vi "XNET Bus Monitor Example.vi"() -> ()   [LabVIEW 2025, in "XNET Bus Monitor Client.lvlib"]
uses:
  XNET Bus Monitor Client.lvlib
  xnet_can_bus_monitor_api_client/RPC Messages/ni_xnet_can_bm_api_FrameFilter.ctl
  xnet_can_bus_monitor_api_client/RPC Messages/ni_xnet_can_bm_api_DirectionFilter.ctl
  Types/GUI.StateVariables.ctl
  Types/GUI.Controls.Refs.ctl
  Types/StreamEngine.QueueRefs.ctl
  Types/StreamEngine.CmdQueueData.ctl
  Types/StreamEngine.CmdQueueData.Cmd.ctl
  Types/SubProcessEngine.QueueRefs.ctl
  Types/SubProcessEngine.CmdQueueData.ctl
  Types/SubProcessEngine.CmdQueueData.Cmd.ctl
  Types/gRPC.ConnectionInfo.ctl
  <vilib>/gRPC/LabVIEW gRPC Library/Shared/grpcId.ctl
  Types/StreamEngine.State.ctl
  Types/SubProcessEngine.State.ctl
  Types/StreamEngine.CmdQueueData.InitialSettings.ctl
  xnet_can_bus_monitor_api_client/RPC Messages/ni_xnet_can_bm_api_StreamBusReply.ctl
  xnet_can_bus_monitor_api_client/RPC Messages/ni_xnet_can_bm_api_CanCommState.ctl
  xnet_can_bus_monitor_api_client/RPC Messages/ni_xnet_can_bm_api_CommState.ctl
  xnet_can_bus_monitor_api_client/RPC Messages/ni_xnet_can_bm_api_LastCommError.ctl
  xnet_can_bus_monitor_api_client/RPC Messages/ni_xnet_can_bm_api_Frame.ctl
  xnet_can_bus_monitor_api_client/RPC Messages/ni_xnet_can_bm_api_ErrorInfo.ctl
  Types/SubProcessEngine.CmdQueueData.Publish.ctl
  Types/StreamEngine.Parameters.ctl
  xnet_can_bus_monitor_api_client/RPC Messages/ni_xnet_can_bm_api_FilterInfo.ctl
  xnet_can_bus_monitor_api_client/RPC Messages/ni_xnet_can_bm_api_PassThruRequest.ctl
  xnet_can_bus_monitor_api_client/RPC Messages/ni_xnet_can_bm_api_SetStreamingFilterRequest.ctl
  <vilib>/Utility/miscctls.llb/LVRowAndColumnUnsignedTypeDef.ctl
  <vilib>/dlg_ctls.llb/Space Constant.vi
  SubVIs/Convert.BusDataArrayToStringArray.vi
  <vilib>/Utility/error.llb/Trim Whitespace.vi
  SubVIs/Convert.TimeToUTCString.vi
  <vilib>/Utility/error.llb/Trim Whitespace One-Sided.vi
  <vilib>/Utility/libraryn.llb/Check if File or Folder Exists.vi
  <vilib>/Utility/libraryn.llb/Get File Extension.vi
  <userlib>/_OpenG.lib/array/array.llb/Sort Array__ogtk.vi
  <userlib>/_OpenG.lib/array/array.llb/Sort 2D Array (String)__ogtk.vi
  xnet_can_bus_monitor_api_client/RPC Service/NI_XNET_CAN_Bus_Monitor_API/Begin NI_XNET_CAN_Bus_Monitor_API StreamBus.vi
  xnet_can_bus_monitor_api_client/RPC Service/NI_XNET_CAN_Bus_Monitor_API/End NI_XNET_CAN_Bus_Monitor_API StreamBus.vi
  xnet_can_bus_monitor_api_client/xnet_can_bus_monitor_api_client.lvlib
  <vilib>/gRPC/LabVIEW gRPC Library/grpc-lvsupport-release.lvlib
panel:
  out "error out":errorcluster
  out "Device":string
  in  "Tab Control":enum32{"Bus Stream", "RAW"}(tab)
  out "Log Status":string
  in  "Direction Filter":T1
  in  "Type Filter":T2
  in  "Reset Filter":bool
  in  "Host Filter":bool
  in  "Filter IDs":string caption="Filter IDs (format = x<ID>, comma separated, ID x0 = Bus Error)"
  in  "Clear History":bool
  out "Table Control":string[][](table)
  in  "Sort By ID":bool
  out "Stream Connected":bool
  out "Bus Status":string
  in  "Log":bool
  in  "Pause":bool
  in  "Extended?":bool
  in  "Identifier":u32 format="%x"
  in  "Raw Bytes":u8[](array[numeric])
  in  "Type":T3(ring)
  out "Error":errorcluster
  in  "Clear Raw":bool
  in  "Send Raw":bool
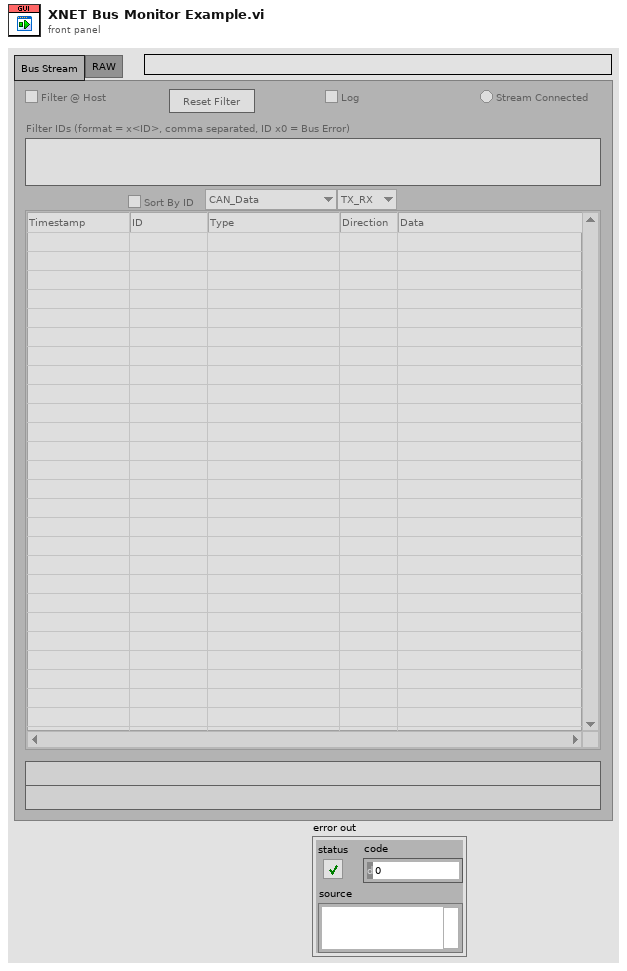
[diagram p1: front panel]
types:
  T1 = typedef "xnet_can_bus_monitor_api_client.lvlib/ni_xnet_can_bm_api_DirectionFilter.ctl" = enum32{"TX_RX", "RX", "TX"}
  T2 = typedef "xnet_can_bus_monitor_api_client.lvlib/ni_xnet_can_bm_api_FrameFilter.ctl" = enum32{"CAN_Data", "CAN_Remote", "CAN_Bus_Error", "CAN_2_Data", "CAN_FD_Data", "CAN_FD_BRS_Data", "J1939_Data", "Delay", "Log_Trigger", "Start_Trigger", "All"}
  T3 = enum16{"CAN Data", "CAN Remote", "CAN Bus Error", "CAN 2.0 Data", "CAN FD Data", "CAN FD+BRS Data", "J1939 Data", "Delay", "Log Trigger", "Start Trigger"}
  T4 = typedef "XNET Bus Monitor Client.lvlib/StreamEngine.CmdQueueData.InitialSettings.ctl" = cluster{"gRPC ID":T5, "Addon":string, "Project Folder":path}
  T5 = typedef "grpc-lvsupport-release.lvlib/grpcId.ctl" = u64
  T6 = typedef "XNET Bus Monitor Client.lvlib/SubProcessEngine.State.ctl" = enum8{"Idle", "Arm", "Process", "Stop", "Exit"}
  T7 = typedef "XNET Bus Monitor Client.lvlib/StreamEngine.State.ctl" = enum8{"Wait", "Start Stream", "Read Stream", "Stop Stream", "Exit"}
  T8 = typedef "XNET Bus Monitor Client.lvlib/GUI.StateVariables.ctl" = cluster{"UI.Refs":T9, "Connected?":bool, "Stream.Qs":T10, "Log Path":path, "gRPC Info":T12}
  T9 = typedef "XNET Bus Monitor Client.lvlib/GUI.Controls.Refs.ctl" = cluster{"Device":refnum<vi>, "Pause":refnum<vi>, "Table Control":refnum<vi>, "Sort By ID":refnum<vi>, "Streaming Connected":refnum<vi>, "Bus Status":refnum<vi>, "Direction Filter":refnum<vi>, "Type Filter":refnum<vi>, "Clear History":refnum<vi>, "Filter IDs":refnum<vi>, "Filter Location":refnum<vi>, "Reset Filter":refnum<vi>, "Log":refnum<vi>, "Type":refnum<vi>, "Extended?":refnum<vi>, "Identifier":refnum<vi>, "Raw Bytes":refnum<vi>, "Send Raw":refnum<vi>, "Clear Raw":refnum<vi>, "Raw Error":refnum<vi>, "Log Status":refnum<vi>}
  T10 = typedef "XNET Bus Monitor Client.lvlib/StreamEngine.QueueRefs.ctl" = cluster{"Cmd":refnum<queue>, "SubProcesses":T11}
  T11 = typedef "XNET Bus Monitor Client.lvlib/SubProcessEngine.QueueRefs.ctl" = cluster{"Process":refnum<queue>, "Log":refnum<queue>}
  T12 = typedef "XNET Bus Monitor Client.lvlib/gRPC.ConnectionInfo.ctl" = cluster{"IP Address":string, "Service Name":string, "Found Port":u64, "ID":T5}
  T13 = typedef "xnet_can_bus_monitor_api_client.lvlib/ni_xnet_can_bm_api_PassThruRequest.ctl" = cluster{"frame":T14}
  T14 = typedef "xnet_can_bus_monitor_api_client.lvlib/ni_xnet_can_bm_api_Frame.ctl" = cluster{"timestamp":dbl, "payload":u8[], "identifier":u32, "frame_type":u32, "extended":bool, "echo":bool}
  T15 = typedef "xnet_can_bus_monitor_api_client.lvlib/ni_xnet_can_bm_api_SetStreamingFilterRequest.ctl" = cluster{"filter_info":T16}
  T16 = typedef "xnet_can_bus_monitor_api_client.lvlib/ni_xnet_can_bm_api_FilterInfo.ctl" = cluster{"filter_ids":u32[], "direction_filter":T1, "frame_filter":T2}
  T17 = typedef "LVRowAndColumnUnsignedTypeDef.ctl" = cluster{"Row":u32, "Column":u32}
  T18 = typedef "xnet_can_bus_monitor_api_client.lvlib/ni_xnet_can_bm_api_StopProcessReply.ctl" = cluster{"stopped":bool, "error":T19}
  T19 = typedef "xnet_can_bus_monitor_api_client.lvlib/ni_xnet_can_bm_api_ErrorInfo.ctl" = errorcluster
  T20 = enum8{"Enabled", "Disabled", "Disabled and Grayed Out"}
  T21 = typedef "xnet_can_bus_monitor_api_client.lvlib/ni_xnet_can_bm_api_PassThruReply.ctl" = cluster{"error":T19}
  T22 = typedef "xnet_can_bus_monitor_api_client.lvlib/ni_xnet_can_bm_api_SetStreamingFilterReply.ctl" = cluster{"error":T19}
  T23 = typedef "xnet_can_bus_monitor_api_client.lvlib/ni_xnet_can_bm_api_ResetStreamingFilterReply.ctl" = cluster{"filter_info":T16, "error":T19}
  T24 = typedef "xnet_can_bus_monitor_api_client.lvlib/ni_xnet_can_bm_api_GetStreamingFilterReply.ctl" = cluster{"filter_info":T16, "error":T19}
  T25 = typedef "XNET Bus Monitor Client.lvlib/SubProcessEngine.CmdQueueData.Publish.ctl" = cluster{"Response Data":T26, "Success":bool}
  T26 = typedef "xnet_can_bus_monitor_api_client.lvlib/ni_xnet_can_bm_api_StreamBusReply.ctl" = cluster{"can_comm_state":T27, "frame":T14[], "error":T19}
  T27 = typedef "xnet_can_bus_monitor_api_client.lvlib/ni_xnet_can_bm_api_CanCommState.ctl" = cluster{"fault_code":i32, "fault":bool, "comm_state":T28, "last_comm_error":T29, "receive_error_counter":u32, "transmit_error_counter":u32, "transceiver_error":bool, "sleep":bool}
  T28 = typedef "xnet_can_bus_monitor_api_client.lvlib/ni_xnet_can_bm_api_CommState.ctl" = enum32{"Error_Active", "Error_Passive", "Bus_Off", "Init"}
  T29 = typedef "xnet_can_bus_monitor_api_client.lvlib/ni_xnet_can_bm_api_LastCommError.ctl" = enum32{"None", "Stuff", "Form", "ACK", "Bit1", "Bit0", "CRC"}
  T30 = typedef "XNET Bus Monitor Client.lvlib/SubProcessEngine.CmdQueueData.ctl" = cluster{"Cmd":T31, "Parameters":variant}
  T31 = typedef "XNET Bus Monitor Client.lvlib/SubProcessEngine.CmdQueueData.Cmd.ctl" = enum16{"Arm", "Publish", "Stop", "Exit"}
  T32 = typedef "XNET Bus Monitor Client.lvlib/StreamEngine.Parameters.ctl" = cluster{"Host Filter":bool, "Filter Parameters":T16, "Sort By ID":bool, "Pause":bool, "Clear History":bool}
  T33 = typedef "XNET Bus Monitor Client.lvlib/StreamEngine.CmdQueueData.ctl" = cluster{"Cmd":T34, "Parameters":variant}
  T34 = typedef "XNET Bus Monitor Client.lvlib/StreamEngine.CmdQueueData.Cmd.ctl" = enum8{"Start Stream", "Stop Stream", "Exit"}
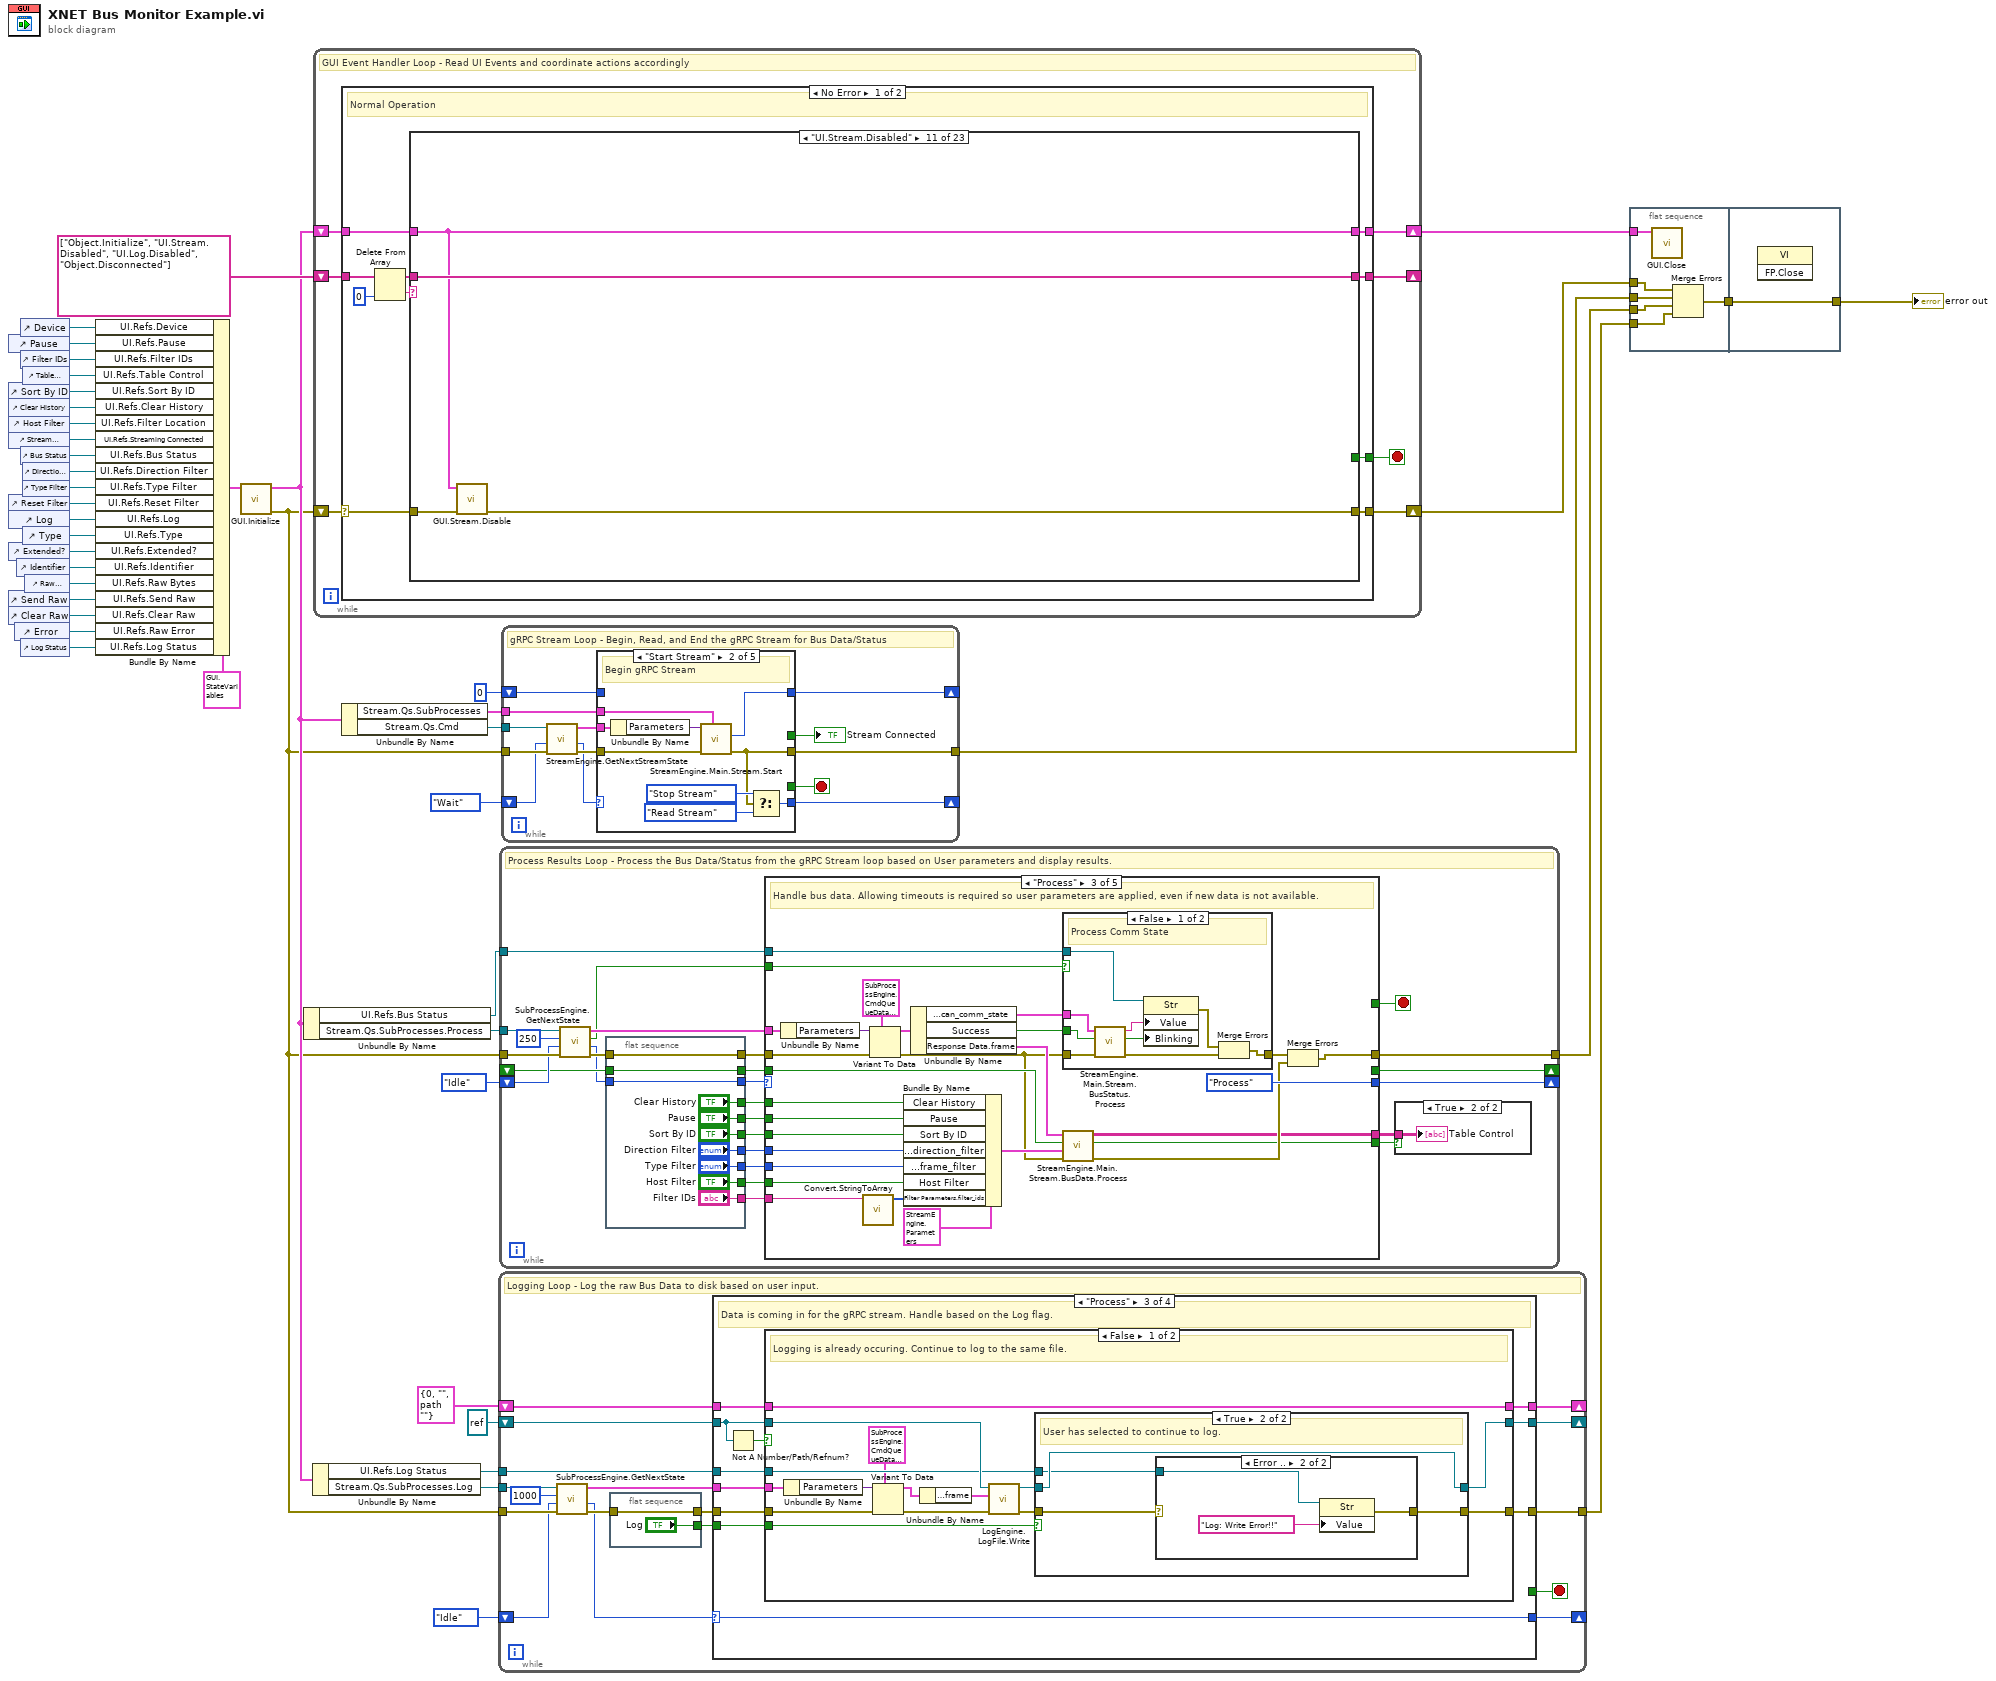
[diagram p0: block diagram]
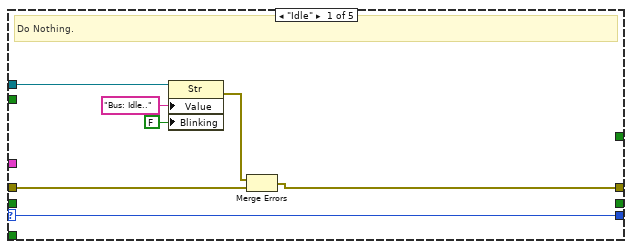
[diagram p3: hidden frame]
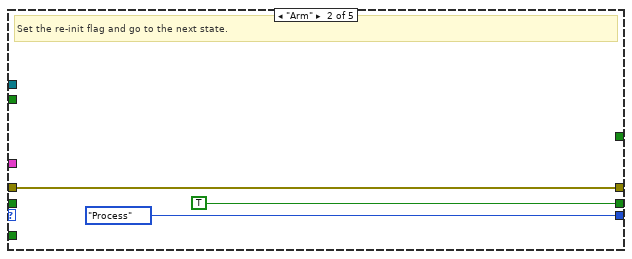
[diagram p4: hidden frame]
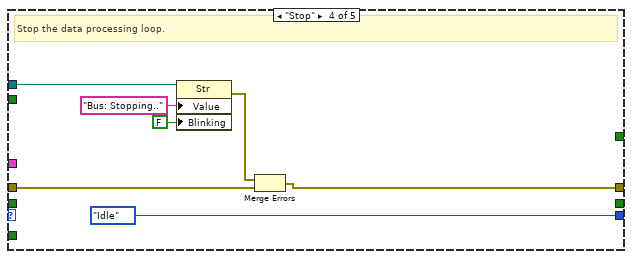
[diagram p6: hidden frame]
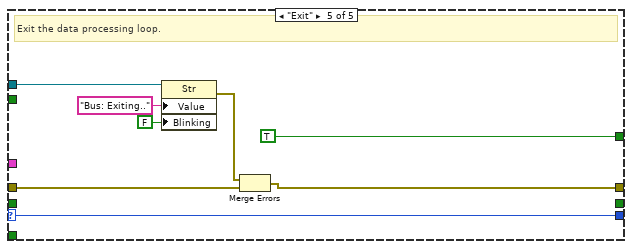
[diagram p7: hidden frame]
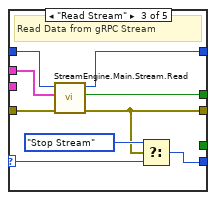
[diagram p9: hidden frame]
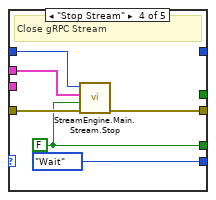
[diagram p10: hidden frame]
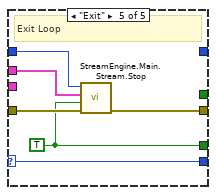
[diagram p11: hidden frame]
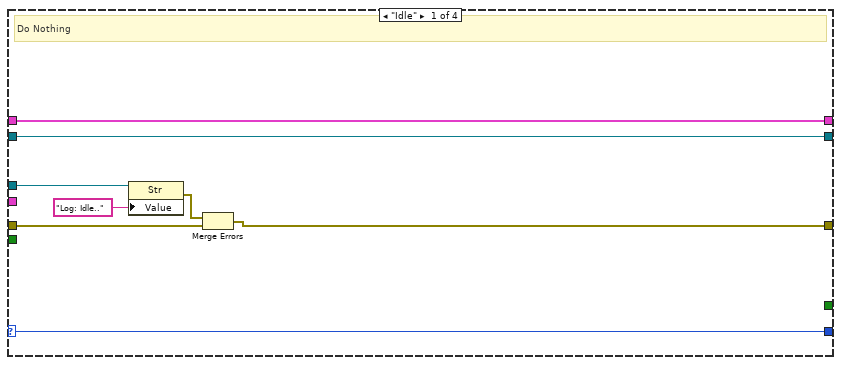
[diagram p12: hidden frame]
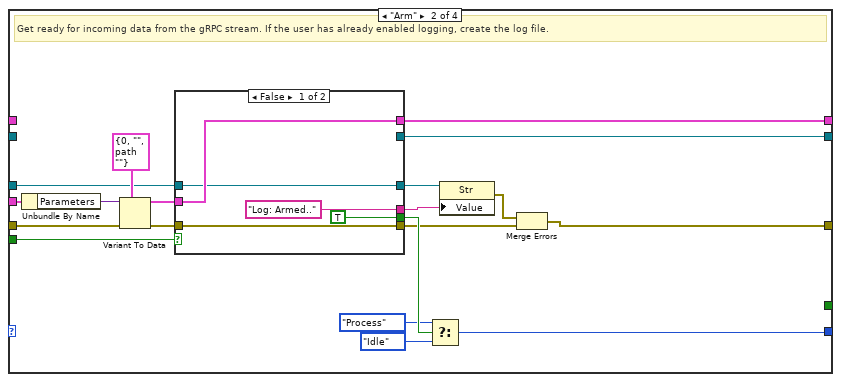
[diagram p13: hidden frame]
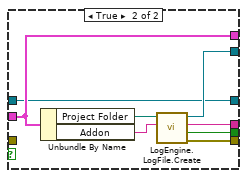
[diagram p14: hidden frame]
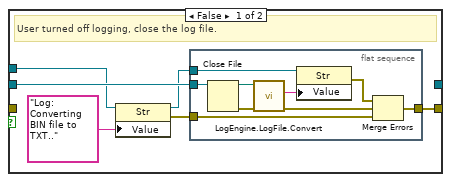
[diagram p15: hidden frame]
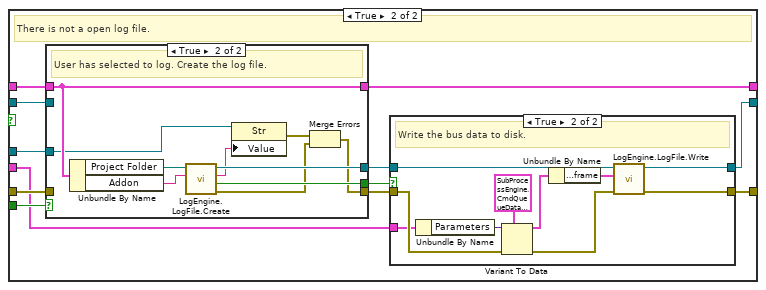
[diagram p17: hidden frame]
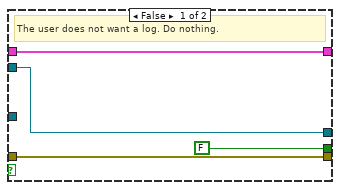
[diagram p19: hidden frame]
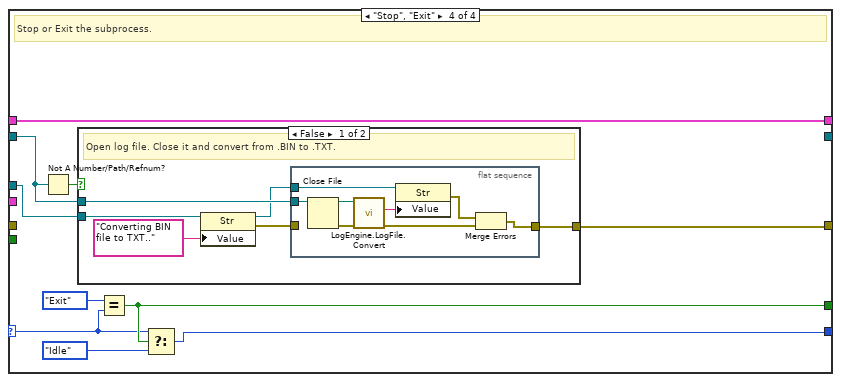
[diagram p20: hidden frame]
diagram:
  n1 = control-ref of="Pause"() -> (w22:refnum<vi>)
  n2 = control-ref of="Sort By ID"() -> (w41:refnum<vi>)
  n3 = control-ref of="Clear History"() -> (w37:refnum<vi>)
  n4 = control-ref of="Host Filter"() -> (w36:refnum<vi>)
  n5 = control-ref of="Stream Connected"() -> (w40:refnum<vi>)
  n6 = control-ref of="Reset Filter"() -> (w35:refnum<vi>)
  n7 = control-ref of="Log"() -> (w34:refnum<vi>)
  n8 = control-ref of="Extended?"() -> (w30:refnum<vi>)
  n9 = control-ref of="Send Raw"() -> (w27:refnum<vi>)
  n10 = control-ref of="Clear Raw"() -> (w28:refnum<vi>)
  n11 = control-ref of="Error"() -> (w29:refnum<vi>)
  n12 = control-ref of="Identifier"() -> (w31:refnum<vi>)
  n13 = control-ref of="Device"() -> (w24:refnum<vi>)
  n14 = control-ref of="Filter IDs"() -> (w38:refnum<vi>)
  n15 = control-ref of="Bus Status"() -> (w39:refnum<vi>)
  n16 = control-ref of="Log Status"() -> (w6:refnum<vi>)
  n17 = control-ref of="Table Control"() -> (w42:refnum<vi>)
  n18 = control-ref of="Direction Filter"() -> (w25:refnum<vi>)
  n19 = control-ref of="Type Filter"() -> (w26:refnum<vi>)
  n20 = control-ref of="Type"() -> (w33:refnum<vi>)
  n21 = control-ref of="Raw Bytes"() -> (w32:refnum<vi>)
  n22 = Bundle By Name(cluster=T8 {"UI.Refs"={"Device"=refnum, "Pause"=refnum, "Table Control"=refnum, "Sort By ID"=refnum, "Streaming Connected"=refnum, "Bus Status"=refnum, "Direction Filter"=refnum, "Type Filter"=refnum, "Clear History"=refnum, "Filter IDs"=refnum, "Filter Location"=refnum, "Reset Filter"=refnum, "Log"=refnum, "Type"=refnum, "Extended?"=refnum, "Identifier"=refnum, "Raw Bytes"=refnum, "Send Raw"=refnum, "Clear Raw"=refnum, "Raw Error"=refnum, "Log Status"=refnum}, "Connected?"=FALSE, "Stream.Qs"={"Cmd"=refnum, "SubProcesses"={"Process"=refnum, "Log"=refnum}}, "Log Path"=path "", "gRPC Info"={"IP Address"="", "Service Name"="", "Found Port"=0, "ID"=0}}, "UI.Refs.Device"=w24, "UI.Refs.Pause"=w22, "UI.Refs.Filter IDs"=w38, "UI.Refs.Table Control"=w42, "UI.Refs.Sort By ID"=w41, "UI.Refs.Clear History"=w37, "UI.Refs.Filter Location"=w36, "UI.Refs.Streaming Connected"=w40, "UI.Refs.Bus Status"=w39, "UI.Refs.Direction Filter"=w25, "UI.Refs.Type Filter"=w26, "UI.Refs.Reset Filter"=w35, "UI.Refs.Log"=w34, "UI.Refs.Type"=w33, "UI.Refs.Extended?"=w30, "UI.Refs.Identifier"=w31, "UI.Refs.Raw Bytes"=w32, "UI.Refs.Send Raw"=w27, "UI.Refs.Clear Raw"=w28, "UI.Refs.Raw Error"=w29, "UI.Refs.Log Status"=w6) -> (w23:T8)
  n23 = call "GUI.Initialize.vi"("State Variables in"=w23) -> ("error out"=w10:errorcluster, "State Variables out"=w13:T8)  [unwired: 9 in]
  n24 = Unbundle By Name(w13) -> ("UI.Refs.Bus Status"=w17:refnum<vi>, "Stream.Qs.SubProcesses.Process"=w18:refnum<queue>)
  n25 = Unbundle By Name(w13) -> ("UI.Refs.Log Status"=w5:refnum<vi>, "Stream.Qs.SubProcesses.Log"=w12:refnum<queue>)
  n26 = while {
    shift-right: [w50] -> _
    shift-left: string[] ["Object.Initialize", "UI.Stream.Disabled", "UI.Log.Disabled", "Object.Disconnected"] -> [w51]
    shift-right: [w48] -> w43
    shift-left: w13 -> [w47]
    shift-right: [w49] -> w8
    shift-left: w10 -> [w46]
    stop <- w52 stop-if-true
    # "GUI Event Handler Loop - Read UI Events and coordinate actions accordingly"
    n27 = case shown="No Error" w46 {
      selector: w46 -> [w53 w402]
      tunnel: [w62 _] -> w52
      tunnel: w51 -> [w60 w406]
      tunnel: [w57 w406] -> w50
      tunnel: [w56 w403] -> w49
      tunnel: [w55 w405] -> w48
      tunnel: w47 -> [w54 w405]
      frame No Error {
        # "Normal Operation"
        n28 = Delete From Array(array=w60, index=0) -> (deleted portion=w59:string, array with subset deleted=w58:string[])  [unwired: 1 in]
        n29 = case shown="\"UI.Stream.Disabled\"" w59 {
          tunnel: [_ _ _ _ _ _ _ _ _ _ _ _ _ _ _ _ _ _ _ _ _ FALSE TRUE] -> w62
          tunnel: [w65 w71 w170 w178 w227 w235 w258 w260 w267 w281 w294 w307 w324 w328 w336 w349 w357 w369 w380 w386 w391 w397 w401] -> w57
          tunnel: w53 -> [w64 w69 w166 w176 w224 w232 w256 w262 w265 w278 w292 w304 w323 w327 w335 w347 w355 w367 w378 w381 w387 w394 w398]
          tunnel: w58 -> [w65 w70 w170 w177 w227 w235 w258 w259 w267 w281 w294 w307 w324 w328 w336 w349 w357 w369 w380 w386 w391 w397 w401]
          tunnel: w54 -> [w63 w66 w169 w174 w225 w229 w255 w263 w264 w280 w293 w306 w322 w326 w333 w348 w356 w368 w379 w385 w390 w393 w399]
          tunnel: [w64 w68 w162 w175 w214 w231 w246 w262 w266 w269 w291 w296 w323 w327 w334 w347 w355 w367 w378 w382 w388 w395 w398] -> w56
          tunnel: [w63 w67 w169 w179 w221 w230 w250 w263 w264 w280 w293 w306 w322 w326 w333 w348 w356 w368 w379 w385 w390 w393 w399] -> w55
          frame Default {
            # "Do nothing."
          }
          frame "" {
            # "Check for new events."
            n30 = event shown="[1] \"Send Raw\": Value Change" {
              selector: _ -> [_ _ _ _ _ _ _ _ _ _]
              dyn-events: _ -> [_ _ _ _ _ _ _ _ _ _]
              timeout: 250 -> [_ _ _ _ _ _ _ _ _ _]
              tunnel: [w73 w78 w87 w99 w110 w119 w129 w142 w151 w158] -> w71
              tunnel: w70 -> [w73 w79 w88 w98 w109 w118 w128 w141 w152 w159]
              tunnel: w69 -> [w75 w80 w89 w100 w111 w120 w130 w143 w155 w161]
              tunnel: [w75 w80 w89 w100 w111 w120 w130 w143 w155 w161] -> w68
              tunnel: [w74 w77 w86 w97 w108 w117 w127 w140 w154 w160] -> w67
              tunnel: w66 -> [w74 w77 w86 w97 w108 w117 w127 w140 w154 w160]
              event Timeout {
                # "No new events to be handled. Do Nothing."
                n31 = event-data() -> ()  [unwired: 2 out]
              }
              event "Send Raw": Value Change {
                # "User entered a new raw message and is ready to Send."
                n32 = event-data() -> ()  [unwired: 2 out]
                n33 = Unbundle By Name(w77) -> ("Connected?"=w76:bool)
                n34 = case shown="True" w76 {
                  tunnel: w79 -> [w81 w83]
                  tunnel: [w81 w82] -> w78
                  frame False {
                  }
                  frame True {
                    n35 = Build Array (concatenate)(w83, string[] ["Raw.Send"]) -> (w82:string[])
                  }
                }
              }
              event "Clear Raw": Value Change {
                # "The user has selected to clear all the values in the Raw tab."
                n36 = event-data() -> ()  [unwired: 2 out]
                n37 = Unbundle By Name(w86) -> ("Connected?"=w85:bool)
                n38 = case shown="True" w85 {
                  tunnel: w88 -> [w90 w92]
                  tunnel: [w90 w91] -> w87
                  frame False {
                  }
                  frame True {
                    n39 = Build Array (concatenate)(w92, string[] ["Raw.Clear"]) -> (w91:string[])
                  }
                }
              }
              event "Filter IDs": Value Change {
                # "The user has changed which IDs to filter. Apply changes."
                n40 = event-data() -> ()  [unwired: 2 out]
                n41 = Unbundle By Name(w97) -> ("Connected?"=w95:bool)
                n42 = local read "Host Filter"() -> (w96:bool)
                n43 = Compound Arithmetic op=AND(invert w96, w95) -> (w94:bool)
                n44 = case shown="False" w94 {
                  tunnel: w98 -> [w101 w105]
                  tunnel: [w102 w104] -> w99
                  frame False {
                    # "Handle filtering on the client/host."
                    n45 = Build Array (concatenate)(w101, "Stream.Table.GoUp") -> (w102:string[])
                  }
                  frame True {
                    # "Send updated filter parameters to Server."
                    n46 = Build Array (concatenate)(w105, string[] ["Stream.Filter.Send", "Stream.Table.GoUp"]) -> (w104:string[])
                  }
                }
              }
              event "Clear History", "Sort By ID": Value Change {
                # "The user has selected to make table changes. The processing loop will handle this but make the table go to the top."
                n47 = event-data() -> ()  [unwired: 2 out]
                n48 = Unbundle By Name(w108) -> ("Connected?"=w107:bool)
                n49 = case shown="True" w107 {
                  tunnel: [w112 w115] -> w110
                  tunnel: w109 -> [w112 w114]
                  frame False {
                  }
                  frame True {
                    n50 = Build Array (concatenate)(w114, "Stream.Table.GoUp") -> (w115:string[])
                  }
                }
              }
              event "Reset Filter": Value Change {
                # "The user has reset which IDs to filter. Apply changes."
                n51 = event-data() -> ()  [unwired: 2 out]
                n52 = Unbundle By Name(w117) -> ("Connected?"=w116:bool)
                n53 = case shown="True" w116 {
                  tunnel: w118 -> [w121 w123]
                  tunnel: [w121 w122] -> w119
                  frame False {
                  }
                  frame True {
                    n54 = Build Array (concatenate)(w123, string[] ["Stream.Filter.Reset", "Stream.Table.GoUp"]) -> (w122:string[])
                  }
                }
              }
              event "Host Filter": Value Change {
                # "The user has changed where filtering happens. Apply changes."
                n55 = event-data() -> ("NewVal"=w125:bool)  [unwired: 1 out]
                n56 = Unbundle By Name(w127) -> ("Connected?"=w126:bool)
                n57 = case shown="True" w126 {
                  tunnel: w128 -> [w131 w134]
                  tunnel: [w131 w133] -> w129
                  tunnel: w125 -> [_ w132]
                  frame False {
                  }
                  frame True {
                    n58 = case shown="True" w132 {
                      tunnel: [string[] ["Stream.Filter.Send", "Stream.Table.GoUp"] string[] ["Stream.Filter.Clear", "Stream.Table.GoUp"]] -> w135
                      frame False {
                      }
                      frame True {
                      }
                    }
                    n59 = Build Array (concatenate)(w134, w135) -> (w133:string[])
                  }
                }
              }
              event "Log": Value Change {
                # "Log loop will handle the logging but force the GUI to latch the configuration while a log session is occuring."
                n60 = event-data() -> ("NewVal"=w138:bool)  [unwired: 1 out]
                n61 = Unbundle By Name(w140) -> ("Connected?"=w139:bool)
                n62 = case shown="True" w139 {
                  tunnel: w141 -> [w144 w147]
                  tunnel: [w144 w146] -> w142
                  tunnel: w138 -> [_ w145]
                  frame False {
                  }
                  frame True {
                    n63 = case shown="False" w145 {
                      tunnel: [string[] ["UI.Log.Disabled"] string[] ["UI.Log.Enabled"]] -> w148
                      frame False {
                      }
                      frame True {
                      }
                    }
                    n64 = Build Array (concatenate)(w147, w148) -> (w146:string[])
                  }
                }
              }
              event Menu Selection (User) {
                # "Queue up the Configure or Exit commands from the run time menu."
                n65 = event-data() -> ("ItemTag"=w153:string)  [unwired: 1 out]
                n66 = Build Array (concatenate)(w152, w153) -> (w151:string[])
              }
              event Panel Close? {
                # "Discard the user panel close and handle nicely."
                n67 = event-data() -> ()  [unwired: 5 out]
                n68 = Build Array (concatenate)(w159, "Object.Exit") -> (w158:string[])
                n69 = event-data("Discard?"=TRUE) -> ()  [unwired: 1 in, 1 out]
              }
            }
          }
          frame "Object.Initialize" {
            # "Initialize the GUI"
            n70 = Unbundle By Name(w169) -> ("UI.Refs.Device"=w164:refnum<vi>, "UI.Refs.Filter Location"=w167:refnum<vi>)
            n71 = property class="Bool (strict)"(reference=w167, error in=w166, "Value"=FALSE) -> (error out=w163:errorcluster)  [unwired: 1 out]
            n72 = local write "Tab Control"(0) -> ()
            n73 = property class="Str"(reference=w164, error in=w163, "Value"="Initializing!!") -> (error out=w162:errorcluster)  [unwired: 1 out]
          }
          frame "Object.Configure" {
            # "Allow the user to select a Port to display"
            n74 = Unbundle By Name(w174) -> ("gRPC Info.ID"=w173:T5)
            n75 = Equal To 0?(x=w173) -> (x = 0?=w172:bool)
            n76 = case shown="True" w172 {
              tunnel: [w181 w201] -> w179
              tunnel: [w180 w200] -> w178
              tunnel: w177 -> [w183 w199]
              tunnel: w176 -> [w187 w196]
              tunnel: [w187 w195] -> w175
              tunnel: w174 -> [w182 w192]
              frame False {
                # "A connection already exists. Ask the user if they want to close it."
                n77 = Two Button Dialog(message="Configuring will close the current session. Continue?", 2:"Yes" ("T button name (\"OK\")")) -> (T button?=w184:bool)  [unwired: 1 in]
                n78 = case shown="True" w184 {
                  tunnel: w183 -> [w188 _]
                  tunnel: w182 -> [w189 w191]
                  tunnel: [w189 w191] -> w181
                  tunnel: [w188 string[] ["Stream.Disable", "UI.Stream.Disabled", "UI.Log.Disabled", "Object.Disconnect", "Object.Disconnected", "Object.Initialize", "Object.Configure"]] -> w180
                  frame False {
                  }
                  frame True {
                  }
                }
              }
              frame True {
                # "No existing connection. Allow user to configure a new connection."
                n79 = call "GUI.ConfigureUI.vi"("error in (no error)"=w196) -> ("error out"=w194:errorcluster, "Log Path out"=w193:path, "Canceled?"=w198:bool, "gRPC Info"=w197:T12)  [unwired: 7 in]
                n80 = case shown="False" w198 {
                  tunnel: w192 -> [w204 w211]
                  tunnel: [w209 w211] -> w201
                  tunnel: [w207 w212] -> w200
                  tunnel: w199 -> [w208 w212]
                  tunnel: w197 -> [w205 _]
                  tunnel: [w203 w210] -> w195
                  tunnel: w194 -> [w203 w210]
                  tunnel: w193 -> [w202 _]
                  frame False {
                    n81 = Bundle By Name(cluster=w204, "gRPC Info"=w205, "Log Path"=w202) -> (w209:T8)
                    n82 = Build Array (concatenate)(w208, string[] ["Object.Initialize", "Stream.Disable", "UI.Stream.Disabled", "Stream.Enable", "UI.Stream.Enabled", "UI.Log.Enabled", "Object.Connected"]) -> (w207:string[])
                  }
                  frame True {
                    # "User canceled"
                  }
                }
              }
            }
          }
          frame "Object.Connected" {
            # "gRPC connected. Update the GUI accordingly."
            n83 = call "GUI.DisableState.Set.vi"("Enable?"=TRUE, "error in (no error)"=w224, "State Variables in"=w225) -> ("error out"=w220:errorcluster, "State Variables out"=w222:T8)  [unwired: 7 in]
            n84 = Unbundle By Name(w222) -> ("UI.Refs.Log"=w216:refnum<vi>, "Log Path"=w217:path, "UI.Refs.Device"=w219:refnum<vi>, "gRPC Info.Service Name"=w218:string)
            n85 = property class="Str"(reference=w219, error in=w220, "Value"=w218) -> (error out=w215:errorcluster)  [unwired: 1 out]
            n86 = call <vilib>:"Is Path and Not Empty.vi"("path"=w217) -> ("Is Path and Not Empty?"=w213:bool)  [unwired: 4 in]
            n87 = property class="Bool (strict)"(reference=w216, error in=w215, "Visible"=w213) -> (error out=w214:errorcluster)  [unwired: 1 out]
            n88 = Bundle By Name(cluster=w222, "Connected?"=TRUE) -> (w221:T8)
          }
          frame "Object.Disconnect" {
            # "Disconnect from the Server."
            n89 = Unbundle By Name(w229) -> ("gRPC Info.ID"=w233:T5)
            n90 = Equal To 0?(x=w233) -> (x = 0?=w234:bool)
            n91 = case shown="False" w234 {
              tunnel: w233 -> [w242 _]
              tunnel: w232 -> [w239 w244]
              tunnel: [w239 w244] -> w231
              frame False {
                n92 = call "NI_XNET_CAN_Bus_Monitor_API StopProcess.vi"("gRPC ID"=w242) -> ("error out"=w237:errorcluster, "Response Data"=w238:T18, "gRPC ID out"=w243:T5)  [unwired: 8 in]
                n93 = call "gRPC.Response.GetError.vi"("error in (no error)"=w237, "Response"=w238) -> ("error out"=w236:errorcluster)  [unwired: 9 in]
                n94 = call "Destroy Client.vi"("gRPC ID"=w243) -> ("error out"=w241:errorcluster)  [unwired: 10 in]
                n95 = Merge Errors(w236, w241) -> (w240:errorcluster)
                n96 = call <vilib>:"Simple Error Handler.vi"("error in (no error)"=w240) -> ()  [unwired: 4 in, 5 out]
              }
              frame True {
              }
            }
            n97 = Bundle By Name(cluster=w229, "gRPC Info"=T12 {"IP Address"="", "Service Name"="", "Found Port"=0, "ID"=0}) -> (w230:T8)
          }
          frame "Object.Disconnected" {
            # "Disconnected from the Server. Update the GUI accordingly."
            n98 = call "GUI.DisableState.Set.vi"("Enable?"=FALSE, "error in (no error)"=w256, "State Variables in"=w255) -> ("error out"=w252:errorcluster, "State Variables out"=w251:T8)  [unwired: 7 in]
            n99 = Unbundle By Name(w251) -> ("UI.Refs.Log"=w248:refnum<vi>, "UI.Refs.Device"=w253:refnum<vi>)
            n100 = property class="Str"(reference=w253, error in=w252, "Value"="Object Disconnected - Configure") -> (error out=w247:errorcluster)  [unwired: 1 out]
            n101 = property class="Bool (strict)"(reference=w248, error in=w247, "Visible"=TRUE ("Value")) -> (error out=w246:errorcluster)  [unwired: 1 out]
            n102 = Bundle By Name(cluster=w251, "Connected?"=FALSE) -> (w250:T8)
          }
          frame "Object.Exit" {
            # "Queue all the commands to cleanly exit."
            n103 = Build Array (concatenate)(w259, string[] ["Stream.Disable", "UI.Stream.Disabled", "UI.Log.Disabled", "Object.Disconnect", "Object.Disconnected", "Stream.Exit", "App.Exit"]) -> (w260:string[])
          }
          frame "UI.Stream.Enabled" {
            n104 = call "GUI.Stream.Enable.vi"("error in (no error)"=w265, "State Variables in"=w264) -> ("error out"=w266:errorcluster)  [unwired: 9 in]
          }
          frame "UI.Log.Enabled" {
            w268 = T20."Disabled and Grayed Out" ("Disabled")
            # "Logging has be enabled. Stop the user from changing filter settings so that the data coming from the Server is the same."
            n105 = Unbundle By Name(w280) -> ("UI.Refs.Type Filter"=w273:refnum<vi>, "UI.Refs.Filter IDs"=w272:refnum<vi>, "UI.Refs.Direction Filter"=w271:refnum<vi>, "UI.Refs.Reset Filter"=w276:refnum<vi>, "UI.Refs.Filter Location"=w279:refnum<vi>)
            n106 = property class="Bool (strict)"(reference=w279, error in=w278, "DisabledEnum"=w268) -> (error out=w277:errorcluster, "Value"=w275:bool)  [unwired: 1 out]
            n107 = Build Array(w273, w272, w271) -> (w270:refnum<vi>[])
            n108 = property class="Bool"(reference=w276, error in=w277, "DisabledEnum"=w268) -> (error out=w274:errorcluster)  [unwired: 1 out]
            n109 = case shown="False" w275 {
              tunnel: w274 -> [w284 w290]
              tunnel: w270 -> [w285 _]
              tunnel: [w283 w290] -> w269
              tunnel: w268 -> [w282 _]
              frame False {
                n110 = for {
                  tunnel: w285 -> [w289] mode=indexing
                  shift-right: [w287] -> w283
                  shift-left: w284 -> [w288]
                  tunnel: w282 -> [w286]
                  n111 = property class="Ctl"(reference=w289, error in=w288, "DisabledEnum"=w286) -> (error out=w287:errorcluster)  [unwired: 1 out]
                }
              }
              frame True {
              }
            }
          }
          frame "UI.Stream.Disabled" {
            n112 = call "GUI.Stream.Disable.vi"("error in (no error)"=w292, "State Variables in"=w293) -> ("error out"=w291:errorcluster)  [unwired: 9 in]
          }
          frame "UI.Log.Disabled" {
            w295 = T20."Enabled" ("Disabled")
            # "Logging has been turned off so re-enable the filter options."
            n113 = Unbundle By Name(w306) -> ("UI.Refs.Type Filter"=w300:refnum<vi>, "UI.Refs.Filter IDs"=w299:refnum<vi>, "UI.Refs.Direction Filter"=w298:refnum<vi>, "UI.Refs.Reset Filter"=w302:refnum<vi>, "UI.Refs.Filter Location"=w305:refnum<vi>)
            n114 = property class="Bool (strict)"(reference=w305, error in=w304, "DisabledEnum"=w295) -> (error out=w303:errorcluster)  [unwired: 1 out]
            n115 = Build Array(w300, w299, w298) -> (w297:refnum<vi>[])
            n116 = property class="Bool"(reference=w302, error in=w303, "DisabledEnum"=w295) -> (error out=w301:errorcluster)  [unwired: 1 out]
            n117 = for {
              tunnel: w297 -> [w311] mode=indexing
              shift-right: [w309] -> w296
              shift-left: w301 -> [w310]
              tunnel: w295 -> [w308]
              n118 = property class="Ctl"(reference=w311, error in=w310, "DisabledEnum"=w308) -> (error out=w309:errorcluster)  [unwired: 1 out]
            }
          }
          frame "Raw.Send" {
            # "Send a raw frame to be put directly on the bus."
            n119 = Bundle By Name(cluster=T13 {"frame"={"timestamp"=0.0, "payload"=[], "identifier"=0, "frame_type"=0, "extended"=FALSE, "echo"=FALSE}} ("Request Data"), "frame.extended"="Extended?", "frame.frame_type"="Type", "frame.identifier"="Identifier", "frame.payload"="Raw Bytes") -> (w316:T13)
            n120 = Unbundle By Name(w322) -> ("gRPC Info.ID"=w315:T5)
            n121 = call "NI_XNET_CAN_Bus_Monitor_API PassThru.vi"("Request Data"=w316, "gRPC ID"=w315) -> ("error out"=w313:errorcluster, "Response Data"=w314:T21)  [unwired: 7 in, 1 out]
            n122 = call "gRPC.Response.GetError.vi"("error in (no error)"=w313, "Response"=w314) -> ("error out"=→"Error":errorcluster)  [unwired: 9 in]
          }
          frame "Raw.Clear" {
            # "Clear the raw bytes GUI."
            n123 = local write "Raw Bytes"(u8[] [] ("Cmd")) -> ()
          }
          frame "Stream.Enable" {
            # "Start the gRPC stream loop."
            n124 = Unbundle By Name(w333) -> ("Stream.Qs"=w332:T10, "gRPC Info.ID"=w331:T5, "gRPC Info.Service Name"=w330:string, "Log Path"=w329:path)
            n125 = call "StreamEngine.StartCmd.Send.vi"("Project Folder"=w329, "error in (no error)"=w335, "Addon"=w330, "gRPC ID"=w331, "Q Refs"=w332) -> ("error out"=w334:errorcluster)  [unwired: 6 in]
          }
          frame "Stream.Filter.Send" {
            # "Send a filter update to the server."
            n126 = local read "Direction Filter"() -> (w345:T1)
            n127 = local read "Type Filter"() -> (w344:T2)
            n128 = local read "Filter IDs"() -> (w346:string)
            n129 = Unbundle By Name(w348) -> ("gRPC Info.ID"=w340:T5)
            n130 = call "Convert.StringToArray.vi"("Filter IDs"=w346) -> ("Filter IDs"=w343:u32[])  [unwired: 10 in]
            n131 = Bundle By Name(cluster=T15 {"filter_info"={"filter_ids"=[], "direction_filter"=enum."TX_RX", "frame_filter"=enum."CAN_Data"}} ("Request Data"), "filter_info.frame_filter"=w344, "filter_info.direction_filter"=w345, "filter_info.filter_ids"=w343) -> (w341:T15)
            n132 = call "NI_XNET_CAN_Bus_Monitor_API SetStreamingFilter.vi"("Request Data"=w341, "gRPC ID"=w340) -> ("error out"=w339:errorcluster, "Response Data"=w337:T22)  [unwired: 7 in, 1 out]
            n133 = call "gRPC.Response.GetError.vi"("error in (no error)"=w339, "Response"=w337) -> ("error out"=w338:errorcluster)  [unwired: 9 in]
            n134 = call <vilib>:"Simple Error Handler.vi"("error in (no error)"=w338) -> ()  [unwired: 4 in, 5 out]
          }
          frame "Stream.Filter.Clear" {
            # "Command the server to clear out the filters."
            n135 = Unbundle By Name(w356) -> ("gRPC Info.ID"=w353:T5)
            n136 = call "NI_XNET_CAN_Bus_Monitor_API SetStreamingFilter.vi"("Request Data"=T15 {"filter_info"={"filter_ids"=[], "direction_filter"=enum."TX_RX", "frame_filter"=enum."CAN_Data"}}, "gRPC ID"=w353) -> ("error out"=w351:errorcluster, "Response Data"=w352:T22)  [unwired: 7 in, 1 out]
            n137 = call "gRPC.Response.GetError.vi"("error in (no error)"=w351, "Response"=w352) -> ("error out"=w350:errorcluster)  [unwired: 9 in]
            n138 = call <vilib>:"Simple Error Handler.vi"("error in (no error)"=w350) -> ()  [unwired: 4 in, 5 out]
          }
          frame "Stream.Filter.Reset" {
            # "Send a command to the server to reset the filter back to the default configuration."
            n139 = Unbundle By Name(w368) -> ("gRPC Info.ID"=w361:T5)
            n140 = call "NI_XNET_CAN_Bus_Monitor_API ResetStreamingFilter.vi"("gRPC ID"=w361) -> ("error out"=w359:errorcluster, "Response Data"=w360:T23)  [unwired: 8 in, 1 out]
            n141 = Unbundle By Name(w360) -> ("filter_info.filter_ids"=w363:u32[], "filter_info.direction_filter"=w365:T1, "filter_info.frame_filter"=w364:T2)
            n142 = call "gRPC.Response.GetError.vi"("error in (no error)"=w359, "Response"=w360) -> ("error out"=w358:errorcluster)  [unwired: 9 in]
            n143 = call <vilib>:"Simple Error Handler.vi"("error in (no error)"=w358) -> ()  [unwired: 4 in, 5 out]
            n144 = local write "Host Filter"(FALSE ("Host Filter")) -> ()
            n145 = call "Convert.ArrayToString.vi"("Filter IDs"=w363) -> ("Filter IDs"=w362:string)  [unwired: 10 in]
            n146 = local write "Filter IDs"(w362) -> ()
            n147 = local write "Direction Filter"(w365) -> ()
            n148 = local write "Type Filter"(w364) -> ()
          }
          frame "Stream.Filter.Read" {
            # "Get the current filter settings from the Server."
            n149 = Unbundle By Name(w379) -> ("gRPC Info.ID"=w373:T5)
            n150 = call "NI_XNET_CAN_Bus_Monitor_API GetStreamingFilter.vi"("gRPC ID"=w373) -> ("error out"=w372:errorcluster, "Response Data"=w371:T24)  [unwired: 8 in, 1 out]
            n151 = Unbundle By Name(w371) -> ("filter_info.filter_ids"=w375:u32[], "filter_info.direction_filter"=w377:T1, "filter_info.frame_filter"=w376:T2)
            n152 = call "gRPC.Response.GetError.vi"("error in (no error)"=w372, "Response"=w371) -> ("error out"=w370:errorcluster)  [unwired: 9 in]
            n153 = call <vilib>:"Simple Error Handler.vi"("error in (no error)"=w370) -> ()  [unwired: 4 in, 5 out]
            n154 = call "Convert.ArrayToString.vi"("Filter IDs"=w375) -> ("Filter IDs"=w374:string)  [unwired: 10 in]
            n155 = local write "Filter IDs"(w374) -> ()
            n156 = local write "Direction Filter"(w377) -> ()
            n157 = local write "Type Filter"(w376) -> ()
          }
          frame "Stream.Table.GoUp" {
            # "Go to the top of the bus table. This is needed for when filters are applied and the user has scrolled down in the list."
            n158 = Unbundle By Name(w385) -> ("UI.Refs.Table Control"=w383:refnum<vi>)
            n159 = property class="Tbl (strict)"(reference=w383, error in=w381, "Index Values"=T17 {"Row"=0, "Column"=0}) -> (error out=w382:errorcluster)  [unwired: 1 out]
          }
          frame "Stream.Disable" {
            # "Stop the gRPC stream to the Server."
            n160 = Unbundle By Name(w390) -> ("Stream.Qs"=w389:T10)
            n161 = call "StreamEngine.StopCmd.Send.vi"("error in (no error)"=w387, "Q Refs"=w389) -> ("error out"=w388:errorcluster)  [unwired: 9 in]
          }
          frame "Stream.Exit" {
            # "Tell the gRPC stream loop to exit."
            n162 = Unbundle By Name(w393) -> ("Stream.Qs"=w392:T10)
            n163 = call "StreamEngine.ExitCmd.Send.vi"("error in (no error)"=w394, "Q Refs"=w392) -> ("error out"=w395:errorcluster)  [unwired: 9 in]
          }
          frame "App.Exit" {
            # "Stop the GUI Event Handler (this) Loop."
          }
        }
      }
      frame Error {
        # "Handle Errors."
        n164 = call <vilib>:"Simple Error Handler.vi"("error in (no error)"=w402) -> ("error out"=w404:errorcluster)  [unwired: 4 in, 4 out]
        n165 = call <vilib>:"Clear Errors.vi"("error in (no error)"=w404) -> ("error out"=w403:errorcluster)  [unwired: 5 in, 1 out]
      }
    }
  }
  n166 = Unbundle By Name(w13) -> ("Stream.Qs.SubProcesses"=w15:T11, "Stream.Qs.Cmd"=w20:refnum<queue>)
  n167 = while {
    tunnel: w12 -> [w423]
    shift-right: [w418] -> _
    shift-left: SubProcessEngine.State."Idle" ("State") -> [w409]
    tunnel: w10 -> [w422]
    shift-right: [w421] -> _
    shift-left: refnum<file> refnum ("Byte Stream File out") -> [w420]
    shift-right: [w416] -> _
    shift-left: T4 {"gRPC ID"=0, "Addon"="", "Project Folder"=path ""} ("cluster") -> [w415]
    tunnel: [w411] -> w7
    tunnel: w5 -> [w410]
    stop <- w417 stop-if-true
    # "Logging Loop - Log the raw Bus Data to disk based on user input."
    n168 = call "SubProcessEngine.GetNextState.vi"("error in (no error)"=w422, "State"=w409, "timeout in ms (5)"=1000, "Q"=w423) -> ("error out"=w413:errorcluster, "State"=w407:T6, "Data"=w419:T30)  [unwired: 4 in, 1 out]
    n169 = flat-sequence {
      tunnel: ["Log"] -> w414
      tunnel: w413 -> [w424]
      tunnel: [w424] -> w412
      frame #0 {
      }
    }
    n170 = case shown="\"Process\"" w407 {
      selector: w407 -> [w432 _ w467 w554]
      tunnel: [w433 w445 w475 _] -> w421
      tunnel: w420 -> [w433 _ w474 w561]
      tunnel: [w427 w437 w476 w553] -> w411
      tunnel: w412 -> [w428 w449 w469 _]
      tunnel: w419 -> [_ w452 w468 _]
      tunnel: [w432 w441 w467 w555] -> w418
      tunnel: [_ _ _ w558] -> w417
      tunnel: [w431 w447 w472 w560] -> w416
      tunnel: w415 -> [w431 _ w473 w560]
      tunnel: w414 -> [_ w440 w471 _]
      tunnel: w410 -> [w430 w435 w466 w559]
      frame "Idle" {
        # "Do Nothing"
        n171 = property class="Str"(reference=w430, "Value"="Log: Idle..") -> (error out=w429:errorcluster)  [unwired: 1 in, 1 out]
        n172 = Merge Errors(w429, w428) -> (w427:errorcluster)
      }
      frame "Arm" {
        # "Get ready for incoming data from the gRPC stream. If the user has already enabled logging, create the log file."
        n173 = Unbundle By Name(w452) -> ("Parameters"=w451:variant)
        n174 = Variant To Data(error in=w449, type=T4 {"gRPC ID"=0, "Addon"="", "Project Folder"=path ""} ("cluster"), Variant=w451) -> (data=w448:T4, error out=w446:errorcluster)
        n175 = case shown="False" w440 {
          tunnel: ["Log: Armed.." ("Status") w463] -> w438
          tunnel: [w457 w462] -> w436
          tunnel: w446 -> [w457 _]
          tunnel: [TRUE ("Continue") w461] -> w444
          tunnel: w448 -> [w455 w460]
          tunnel: [w455 w460] -> w447
          tunnel: [_ w459] -> w445
          tunnel: w435 -> [w453 w458]
          tunnel: [w453 w458] -> w434
          frame False {
          }
          frame True {
            n176 = Unbundle By Name(w460) -> ("Project Folder"=w465:path, "Addon"=w464:string)
            n177 = call "LogEngine.LogFile.Create.vi"("Port"=w464, "Project Folder"=w465) -> ("error out"=w462:errorcluster, "Continue"=w461:bool, "Status"=w463:string, "Byte Stream File out"=w459:refnum<file>)  [unwired: 6 in]
          }
        }
        n178 = Select(t=SubProcessEngine.State."Process" ("State"), s=w444, f=SubProcessEngine.State."Idle") -> (s? t:f=w441:T6)
        n179 = property class="Str"(reference=w434, "Value"=w438) -> (error out=w439:errorcluster)  [unwired: 1 in, 1 out]
        n180 = Merge Errors(w439, w436) -> (w437:errorcluster)
      }
      frame "Process" {
        # "Data is coming in for the gRPC stream. Handle based on the Log flag."
        n181 = Not A Number/Path/Refnum?(number/path/refnum=w474) -> (NaN/Path/Refnum?=w470:bool)
        n182 = case shown="False" w470 {
          tunnel: [w478 w515] -> w476
          tunnel: [w479 w524] -> w475
          tunnel: w474 -> [w489 w523]
          tunnel: w473 -> [w491 w521]
          tunnel: [w491 w520] -> w472
          tunnel: w471 -> [w482 w519]
          tunnel: w469 -> [w490 w518]
          tunnel: w468 -> [w484 w517]
          tunnel: w466 -> [w480 w516]
          frame False {
            # "Logging is already occuring. Continue to log to the same file."
            n183 = Unbundle By Name(w484) -> ("Parameters"=w487:variant)
            n184 = Variant To Data(error in=w490, type=T25 {"Response Data"={"can_comm_state"={"fault_code"=0, "fault"=FALSE, "comm_state"=enum."Error_Active", "last_comm_error"=enum."None", "receive_error_counter"=0, "transmit_error_counter"=0, "transceiver_error"=FALSE, "sleep"=FALSE}, "frame"=[], "error"={"status"=FALSE, "code"=0, "source"=""}}, "Success"=FALSE} ("cluster"), Variant=w487) -> (data=w486:T25, error out=w488:errorcluster)
            n185 = Unbundle By Name(w486) -> ("Response Data.frame"=w485:T14[])
            n186 = call "LogEngine.LogFile.Write.vi"("error in (no error)"=w488, "Data"=w485, "Byte Stream File in"=w489) -> ("error out"=w481:errorcluster, "Byte Stream File out"=w483:refnum<file>)  [unwired: 7 in]
            n187 = case shown="True" w482 {
              tunnel: w483 -> [w497 w510]
              tunnel: [w493 w507] -> w478
              tunnel: w480 -> [w496 w509]
              tunnel: w481 -> [_ w508]
              tunnel: [_ w510] -> w479
              frame False {
                # "User turned off logging, close the log file."
                n188 = property class="Str"(reference=w496, "Value"="Log: Converting BIN file to TXT..") -> (reference out=w494:refnum<vi>, error out=w492:errorcluster)  [unwired: 1 in]
                n189 = flat-sequence {
                  tunnel: w497 -> [w506]
                  tunnel: w494 -> [w502]
                  tunnel: [w500] -> w493
                  tunnel: w492 -> [w498]
                  frame #0 {
                    n190 = Close File(refnum=w506) -> (path=w505:path, error out=w504:errorcluster)  [unwired: 1 in]
                    n191 = call "LogEngine.LogFile.Convert.vi"("error in (no error)"=w504, "path"=w505) -> ("error out"=w499:errorcluster, "Status"=w501:string)  [unwired: 8 in]
                    n192 = property class="Str"(reference=w502, "Value"=w501) -> (error out=w503:errorcluster)  [unwired: 1 in, 1 out]
                    n193 = Merge Errors(w503, w499, w498) -> (w500:errorcluster)
                  }
                }
              }
              frame True {
                # "User has selected to continue to log."
                n194 = case shown="Error .." w508 {
                  selector: w508 -> [w511 _]
                  tunnel: w509 -> [_ w514]
                  tunnel: [w511 w512] -> w507
                  frame No Error {
                  }
                  frame Error {
                    n195 = property class="Str"(reference=w514, "Value"="Log: Write Error!!") -> (error out=w512:errorcluster)  [unwired: 1 in, 1 out]
                  }
                }
              }
            }
          }
          frame True {
            # "There is not a open log file."
            n196 = case shown="True" w519 {
              tunnel: [w541 w543] -> w526
              tunnel: [w542 w550] -> w525
              tunnel: w523 -> [w542 _]
              tunnel: [FALSE ("Continue") w549] -> w522
              tunnel: w518 -> [w541 _]
              tunnel: w521 -> [w540 w548]
              tunnel: [w540 w548] -> w520
              tunnel: w516 -> [_ w546]
              frame False {
                # "The user does not want a log. Do nothing."
              }
              frame True {
                # "User has selected to log. Create the log file."
                n197 = Unbundle By Name(w548) -> ("Project Folder"=w552:path, "Addon"=w551:string)
                n198 = call "LogEngine.LogFile.Create.vi"("Port"=w551, "Project Folder"=w552) -> ("error out"=w544:errorcluster, "Continue"=w549:bool, "Status"=w545:string, "Byte Stream File out"=w550:refnum<file>)  [unwired: 6 in]
                n199 = property class="Str"(reference=w546, "Value"=w545) -> (error out=w547:errorcluster)  [unwired: 1 in, 1 out]
                n200 = Merge Errors(w547, w544) -> (w543:errorcluster)
              }
            }
            n201 = case shown="True" w522 {
              tunnel: w526 -> [w527 w534]
              tunnel: w525 -> [w528 w538]
              tunnel: [w527 w537] -> w515
              tunnel: [w528 w536] -> w524
              tunnel: w517 -> [_ w533]
              frame False {
                # "Do nothing."
              }
              frame True {
                # "Write the bus data to disk."
                n202 = Unbundle By Name(w533) -> ("Parameters"=w532:variant)
                n203 = Variant To Data(error in=w534, type=T25 {"Response Data"={"can_comm_state"={"fault_code"=0, "fault"=FALSE, "comm_state"=enum."Error_Active", "last_comm_error"=enum."None", "receive_error_counter"=0, "transmit_error_counter"=0, "transceiver_error"=FALSE, "sleep"=FALSE}, "frame"=[], "error"={"status"=FALSE, "code"=0, "source"=""}}, "Success"=FALSE} ("cluster"), Variant=w532) -> (data=w531:T25, error out=w535:errorcluster)
                n204 = Unbundle By Name(w531) -> ("Response Data.frame"=w530:T14[])
                n205 = call "LogEngine.LogFile.Write.vi"("error in (no error)"=w535, "Data"=w530, "Byte Stream File in"=w538) -> ("error out"=w537:errorcluster, "Byte Stream File out"=w536:refnum<file>)  [unwired: 7 in]
              }
            }
          }
        }
      }
      frame "Stop", "Exit" {
        # "Stop or Exit the subprocess."
        n206 = Not A Number/Path/Refnum?(number/path/refnum=w561) -> (NaN/Path/Refnum?=w562:bool)
        n207 = case shown="False" w562 {
          tunnel: w561 -> [w568 _]
          tunnel: w559 -> [w567 _]
          tunnel: [w564 _] -> w553
          frame False {
            # "Open log file. Close it and convert from .BIN to .TXT."
            n208 = property class="Str"(reference=w567, "Value"="Converting BIN file to TXT..") -> (reference out=w565:refnum<vi>, error out=w563:errorcluster)  [unwired: 1 in]
            n209 = flat-sequence {
              tunnel: w568 -> [w575]
              tunnel: w565 -> [w572]
              tunnel: [w571] -> w564
              tunnel: w563 -> [_]
              frame #0 {
                n210 = Close File(refnum=w575) -> (path=w570:path, error out=w569:errorcluster)  [unwired: 1 in]
                n211 = call "LogEngine.LogFile.Convert.vi"("error in (no error)"=w569, "path"=w570) -> ("error out"=w573:errorcluster, "Status"=w576:string)  [unwired: 8 in]
                n212 = property class="Str"(reference=w572, "Value"=w576) -> (error out=w574:errorcluster)  [unwired: 1 in, 1 out]
                n213 = Merge Errors(w574, w573) -> (w571:errorcluster)
              }
            }
          }
          frame True {
            # "No open log file. Do nothing."
          }
        }
        n214 = Equal?(x=SubProcessEngine.State."Exit", y=w554) -> (x = y?=w558:bool)
        n215 = Select(t=w554, s=w558, f=SubProcessEngine.State."Idle" ("x")) -> (s? t:f=w555:T6)
      }
    }
  }
  n216 = while {
    tunnel: w18 -> [w600]
    tunnel: w17 -> [w602]
    tunnel: [w601] -> w9
    shift-right: [w599] -> _
    shift-left: SubProcessEngine.State."Idle" ("State") -> [w594]
    tunnel: w10 -> [w598]
    shift-right: [w596] -> _
    shift-left: _ -> [w582]
    stop <- w595 stop-if-true
    # "Process Results Loop - Process the Bus Data/Status from the gRPC Stream loop based on User parameters and display results."
    n217 = call "SubProcessEngine.GetNextState.vi"("error in (no error)"=w598, "State"=w594, "timeout in ms (5)"=250, "Q"=w600) -> ("error out"=w584:errorcluster, "State"=w580:T6, "timed out?"=w593:bool, "Data"=w597:T30)  [unwired: 4 in]
    n218 = flat-sequence {
      tunnel: ["Pause"] -> w591
      tunnel: ["Type Filter"] -> w590
      tunnel: ["Direction Filter"] -> w589
      tunnel: ["Host Filter"] -> w588
      tunnel: ["Filter IDs"] -> w587
      tunnel: ["Clear History"] -> w586
      tunnel: ["Sort By ID"] -> w585
      tunnel: w584 -> [w606]
      tunnel: [w606] -> w583
      tunnel: w582 -> [w605]
      tunnel: [w605] -> w581
      tunnel: w580 -> [w604]
      tunnel: [w604] -> w579
      frame #0 {
      }
    }
    n219 = case shown="\"Process\"" w579 {
      selector: w579 -> [w620 _ _ _ w676]
      tunnel: w602 -> [w616 _ w651 w667 w671]
      tunnel: [w614 w621 w633 w662 w669] -> w601
      tunnel: [w620 SubProcessEngine.State."Process" ("State") SubProcessEngine.State."Process" ("State") SubProcessEngine.State."Idle" ("State") w676] -> w599
      tunnel: w583 -> [w615 w621 w647 w664 w670]
      tunnel: w597 -> [_ _ w649 _ _]
      tunnel: [_ TRUE _ _ _] -> w596
      tunnel: w581 -> [_ _ w637 _ _]
      tunnel: [_ _ _ _ TRUE] -> w595
      tunnel: w593 -> [_ _ w643 _ _]
      tunnel: w591 -> [_ _ w632 _ _]
      tunnel: w590 -> [_ _ w631 _ _]
      tunnel: w589 -> [_ _ w630 _ _]
      tunnel: w588 -> [_ _ w629 _ _]
      tunnel: w587 -> [_ _ w628 _ _]
      tunnel: w586 -> [_ _ w627 _ _]
      tunnel: w585 -> [_ _ w626 _ _]
      tunnel: [_ _ w625 _ _] -> w578
      tunnel: [_ _ w624 _ _] -> w577
      frame "Idle" {
        # "Do Nothing."
        n220 = property class="Str"(reference=w616, "Value"="Bus: Idle..", "Blinking"=FALSE) -> (error out=w617:errorcluster)  [unwired: 1 in, 1 out]
        n221 = Merge Errors(w617, w615) -> (w614:errorcluster)
      }
      frame "Arm" {
        # "Set the re-init flag and go to the next state."
      }
      frame "Process" {
        # "Handle bus data. Allowing timeouts is required so user parameters are applied, even if new data is not available."
        n222 = Unbundle By Name(w649) -> ("Parameters"=w648:variant)
        n223 = call "Convert.StringToArray.vi"("Filter IDs"=w628) -> ("Filter IDs"=w641:u32[])  [unwired: 10 in]
        n224 = Variant To Data(error in=w647, type=T25 {"Response Data"={"can_comm_state"={"fault_code"=0, "fault"=FALSE, "comm_state"=enum."Error_Active", "last_comm_error"=enum."None", "receive_error_counter"=0, "transmit_error_counter"=0, "transceiver_error"=FALSE, "sleep"=FALSE}, "frame"=[], "error"={"status"=FALSE, "code"=0, "source"=""}}, "Success"=FALSE} ("cluster"), Variant=w648) -> (data=w646:T25, error out=w636:errorcluster)
        n225 = Bundle By Name(cluster=T32 {"Host Filter"=FALSE, "Filter Parameters"={"filter_ids"=[], "direction_filter"=enum."TX_RX", "frame_filter"=enum."CAN_Data"}, "Sort By ID"=FALSE, "Pause"=FALSE, "Clear History"=FALSE} ("Host Parameters"), "Clear History"=w627, "Pause"=w632, "Sort By ID"=w626, "Filter Parameters.direction_filter"=w630, "Filter Parameters.frame_filter"=w631, "Host Filter"=w629, "Filter Parameters.filter_ids"=w641) -> (w638:T32)
        n226 = Unbundle By Name(w646) -> ("Response Data.can_comm_state"=w644:T27, "Success"=w639:bool, "Response Data.frame"=w645:T14[])
        n227 = case shown="False" w643 {
          tunnel: w651 -> [w660 _]
          tunnel: [w656 w661] -> w635
          tunnel: w644 -> [w655 _]
          tunnel: w639 -> [w653 _]
          tunnel: w636 -> [w652 w661]
          frame False {
            # "Process Comm State"
            n228 = call "StreamEngine.Main.Stream.BusStatus.Process.vi"("error in (no error)"=w652, "Stream Connection"=w653, "State"=w655) -> ("error out"=w657:errorcluster, "Warning"=w659:bool, "State"=w654:string)  [unwired: 6 in]
            n229 = property class="Str"(reference=w660, "Value"=w654, "Blinking"=w659) -> (error out=w658:errorcluster)  [unwired: 1 in, 1 out]
            n230 = Merge Errors(w658, w657) -> (w656:errorcluster)
          }
          frame True {
            # "Timeout. Do nothing."
          }
        }
        n231 = call "StreamEngine.Main.Stream.BusData.Process.vi"("error in (no error)"=w636, "Host Parameters"=w638, "Init?"=w637, "frame"=w645) -> ("error out"=w634:errorcluster, "Table Update"=w625:bool, "Table"=w624:string[][])  [unwired: 5 in]
        n232 = Merge Errors(w635, w634) -> (w633:errorcluster)
      }
      frame "Stop" {
        # "Stop the data processing loop."
        n233 = property class="Str"(reference=w667, "Value"="Bus: Stopping..", "Blinking"=FALSE) -> (error out=w663:errorcluster)  [unwired: 1 in, 1 out]
        n234 = Merge Errors(w663, w664) -> (w662:errorcluster)
      }
      frame "Exit" {
        # "Exit the data processing loop."
        n235 = property class="Str"(reference=w671, "Value"="Bus: Exiting..", "Blinking"=FALSE) -> (error out=w672:errorcluster)  [unwired: 1 in, 1 out]
        n236 = Merge Errors(w672, w670) -> (w669:errorcluster)
      }
    }
    n237 = case shown="True" w578 {
      tunnel: w577 -> [_ w603]
      frame False {
      }
      frame True {
        "Table Control" <- w603
      }
    }
  }
  n238 = while {
    shift-right: [w686] -> _
    shift-left: StreamEngine.State."Wait" -> [w678]
    tunnel: w10 -> [w687]
    shift-right: [w685] -> _
    shift-left: T5 0 ("Call ID") -> [w684]
    tunnel: w20 -> [w682]
    tunnel: [w681] -> w19
    tunnel: w15 -> [w679]
    stop <- w683 stop-if-true
    # "gRPC Stream Loop - Begin, Read, and End the gRPC Stream for Bus Data/Status"
    n239 = call "StreamEngine.GetNextStreamState.vi"("error in (no error)"=w687, "Bus State"=w678, "Cmd Q"=w682) -> ("error out"=w688:errorcluster, "Bus State"=w677:T7, "Command Cluster"=w689:T33)  [unwired: 5 in, 1 out]
    n240 = case shown="\"Start Stream\"" w677 {
      selector: w677 -> [w690 _ w708 _ w719]
      tunnel: w688 -> [w691 w694 w705 w714 w721]
      tunnel: w689 -> [_ w697 _ _ _]
      tunnel: [w691 w695 w703 w712 w718] -> w681
      tunnel: [_ w696 w704 _ _] -> w685
      tunnel: w684 -> [_ _ w706 w713 w720]
      tunnel: [w690 w698 w707 StreamEngine.State."Wait" w719] -> w686
      tunnel: [_ _ _ w711 w717] -> w683
      tunnel: [_ _ w702 _ _] -> w680
      tunnel: w679 -> [_ w693 w701 w710 w716]
      frame "Wait", Default {
        # "Do Nothing"
      }
      frame "Start Stream" {
        # "Begin gRPC Stream"
        n241 = Unbundle By Name(w697) -> ("Parameters"=w692:variant)
        n242 = call "StreamEngine.Main.Stream.Start.vi"("Stream.Qs.SubProcesses"=w693, "error in (no error)"=w694, "Parameters"=w692) -> ("error out"=w695:errorcluster, "Stream Ref"=w696:T5)  [unwired: 6 in, 1 out]
        n243 = Select(t=StreamEngine.State."Stop Stream", s=w695, f=StreamEngine.State."Read Stream") -> (s? t:f=w698:T7)
      }
      frame "Read Stream" {
        # "Read Data from gRPC Stream"
        n244 = call "StreamEngine.Main.Stream.Read.vi"("error in (no error)"=w705, "SubProcesses"=w701, "gRPC ID"=w706) -> ("error out"=w703:errorcluster, "Success"=w702:bool, "gRPC ID out"=w704:T5)  [unwired: 6 in]
        n245 = Select(t=StreamEngine.State."Stop Stream", s=w703, f=w708) -> (s? t:f=w707:T7)
      }
      frame "Stop Stream" {
        w711 = FALSE ("Exit?")
        # "Close gRPC Stream"
        n246 = call "StreamEngine.Main.Stream.Stop.vi"("error in (no error)"=w714, "Exit?"=w711, "Stream.Qs.SubProcesses"=w710, "Stream Ref"=w713) -> ("error out"=w712:errorcluster)  [unwired: 7 in]
      }
      frame "Exit" {
        w717 = TRUE
        # "Exit Loop"
        n247 = call "StreamEngine.Main.Stream.Stop.vi"("error in (no error)"=w721, "Exit?"=w717, "Stream.Qs.SubProcesses"=w716, "Stream Ref"=w720) -> ("error out"=w718:errorcluster)  [unwired: 7 in]
      }
    }
    "Stream Connected" <- w680
  }
  n248 = flat-sequence {
    tunnel: w43 -> [w727]
    tunnel: w19 -> [w725]
    tunnel: w9 -> [w724]
    tunnel: w8 -> [w726]
    tunnel: w7 -> [w723]
    tunnel: [w722] -> w1
    tunnel: [w728] -> w2
    tunnel: w1 -> [w728]
    frame #0 {
      n249 = call "GUI.Close.vi"("State Variables in"=w727) -> ()  [unwired: 11 in]
      n250 = Merge Errors(w726, w725, w724, w723) -> (w722:errorcluster)
    }
    frame #1 {
      n251 = invoke class="VI" method="FP.Close"() -> ()  [unwired: 3 in, 3 out]
    }
  }
  "error out" <- w2
